vi "SysDef.SimpleLoad.vi"(7 "Overwrite Existing?":bool=TRUE, 8 "error in (no error)":errorcluster, 10 "Path":path, 11 "NodeID":u64) -> (0 "error out":errorcluster, 3 "NodeID out":u64)   [LabVIEW 2015, in "System Definition Utilities.lvlib"]
uses:
  System Definition Utilities.lvlib
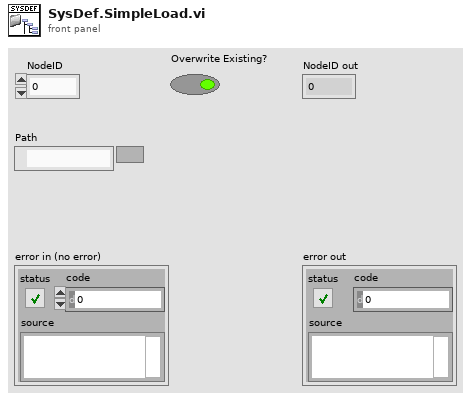
[diagram p1: front panel]
types:
  T1 = typedef "System Definition Utilities.lvlib/SysDef.Export.ctl" = cluster{"Version":string, "Tree":T2[]}
  T2 = typedef "System Definition Utilities.lvlib/TreeItem.ctl" = cluster{"Item Info":T3, "Parent Path":string[], "Properties":T8[]}
  T3 = typedef "System Definition Utilities.lvlib/TreeItem.Info.ctl" = cluster{"Name":string, "Description":string, "GUID":string, "Is Channel":bool, "Channel":T4, "Is Waveform":bool, "Waveform":T6}
  T4 = typedef "Custom Device API.lvlib/Custom Device Channel.ctl" = cluster{"Type":T5, "Units":string, "Default Value":dbl, "Faultable":bool, "Scalable":bool}
  T5 = typedef "Custom Device API.lvlib/Custom Device Channel Type.ctl" = enum16{"Input", "Output"}
  T6 = typedef "Custom Device API.lvlib/Custom Device Waveform.ctl" = cluster{"Data Type":T7, "Units":string}
  T7 = typedef "Custom Device API.lvlib/Custom Device Waveform DataType.ctl" = enum16{"Double", "Complex Double"}
  T8 = typedef "System Definition Utilities.lvlib/TreeItem.Property.ctl" = cluster{"Name":string, "Type":i32, "Value":variant}
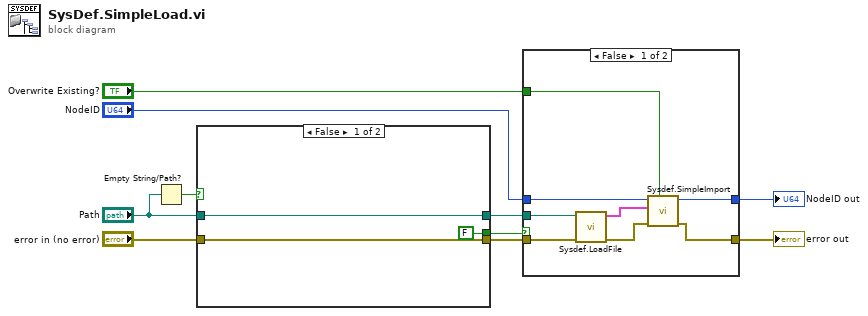
[diagram p0: block diagram]
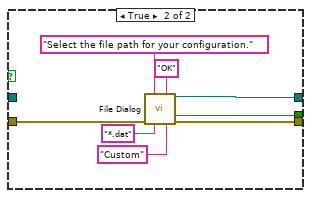
[diagram p2: hidden frame]
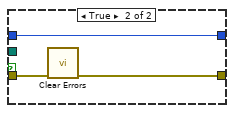
[diagram p3: hidden frame]
diagram:
  n1 = Empty String/Path?(string/path="Path") -> (empty?=w7:bool)
  n2 = case shown="False" w7 {
    tunnel: [FALSE ("cancelled") w17] -> w10
    tunnel: [w11 w16] -> w9
    tunnel: [w12 w15] -> w8
    tunnel: "error in (no error)" -> [w11 w14]
    tunnel: "Path" -> [w12 _]
    frame False {
    }
    frame True {
      n3 = call "File Dialog"("prompt"="Select the file path for your configuration.", "button label"="OK", "error in"=w14, "pattern (all files)"="*.dat", "pattern label"="Custom") -> ("selected path"=w15:path, "cancelled"=w17:bool, "error out"=w16:errorcluster)  [unwired: 7 in, 1 out]
    }
  }
  n4 = case shown="False" w10 {
    tunnel: [w25 w31] -> w3
    tunnel: w9 -> [w27 w32]
    tunnel: w8 -> [w26 _]
    tunnel: "NodeID" -> [w24 w30]
    tunnel: [w23 w30] -> w2
    tunnel: "Overwrite Existing?" -> [w22 _]
    frame False {
      n5 = call "Sysdef.LoadFile.vi"("error in (no error)"=w27, "Path in"=w26) -> ("error out"=w28:errorcluster, "SysDef"=w29:T1)  [unwired: 8 in]
      n6 = call "Sysdef.SimpleImport.vi"("Overwrite Existing?"=w22, "error in (no error)"=w28, "SysDef"=w29, "NodeID"=w24) -> ("error out"=w25:errorcluster, "NodeID out"=w23:u64)  [unwired: 6 in]
    }
    frame True {
      n7 = call <vilib>:"Clear Errors.vi"("error in (no error)"=w32) -> ("error out"=w31:errorcluster)  [unwired: 5 in, 1 out]
    }
  }
  "error out" <- w3
  "NodeID out" <- w2
